vi "PWM舵机驱动实验--基于EIO节点.vi"() -> ()   [LabVIEW 2011]
uses:
  <vilib>/STM32_DriverVI_Interface_F4/PWM-EIO/PWM_Control_F4.ctl
  <vilib>/eio/EIO_TerminalDirection.ctl
  D:/National Instruments/LabVIEW 2011/Targets/Keil/Embedded/RealView/Generic/My_ARM_Starter_Board_F4/STM32_DriverVI_Interface/PWM-EIO/PWM_Channel_16_F4.ctl
  <vilib>/STM32_DriverVI_Interface_F4/Timer/TIM4_Group_Pins_F4.ctl
  <vilib>/STM32_DriverVI_Interface_F4/Timer/TIM4_Channels_Pin_Map_F4.ctl
  <vilib>/STM32_DriverVI_Interface_F4/Timer/TimerX Init_F4.vi
  <vilib>/STM32_DriverVI_Interface_F4/Timer/TIM4 Init_F4.vi
  <vilib>/STM32_DriverVI_Interface_F4/Timer/TimerX Channel Pin Map.vi
  <vilib>/STM32_DriverVI_Interface_F4/Timer/TIM4 Channel Pin Map_F4.vi
  <vilib>/STM32_DriverVI_Interface_F4/Timer/TimerX PWM Mode Set_F4.vi
  <vilib>/STM32_DriverVI_Interface_F4/Timer/TIM4 PWM Mode Set_F4.vi
  <vilib>/STM32_DriverVI_Interface_F4/Timer/TimerX PWM Permit_UnPermit_F4.vi
  <vilib>/STM32_DriverVI_Interface_F4/Timer/TIM4 PWM Permit_UnPermit_F4.vi
  <vilib>/STM32_DriverVI_Interface_F4/Timer/TimerX Int Enable_Disable_F4.vi
  <vilib>/STM32_DriverVI_Interface_F4/Timer/TIM4 Int Enable_Disable_F4.vi
  <vilib>/STM32_DriverVI_Interface_F4/Timer/TimerX PWM Update Duty_F4.vi
  <vilib>/STM32_DriverVI_Interface_F4/Timer/TIM4_PWM_Update_Duty_F4.vi
  <vilib>/eio/EIONode/EIONode.xnode
  <vilib>/STM32_DriverVI_Interface_F4/Timer/TIM5_Channels_Pin_Map_F4.ctl
  <vilib>/STM32_DriverVI_Interface_F4/Timer/TIM5_Group_Pins_F4.ctl
  <vilib>/STM32_DriverVI_Interface_F4/Timer/TIM5 Int Enable_Disable_F4.vi
  <vilib>/STM32_DriverVI_Interface_F4/Timer/TIM5_PWM_Update_Duty_F4.vi
  <vilib>/STM32_DriverVI_Interface_F4/Timer/TIM5 Init_F4.vi
  <vilib>/STM32_DriverVI_Interface_F4/Timer/TIM5 Channel Pin Map_F4.vi
  <vilib>/STM32_DriverVI_Interface_F4/Timer/TIM5 PWM Mode Set_F4.vi
  <vilib>/STM32_DriverVI_Interface_F4/Timer/TIM5 PWM Permit_UnPermit_F4.vi
  <vilib>/STM32_DriverVI_Interface_F4/Timer/TIM3_Channels_Pin_Map_F4.ctl
  <vilib>/STM32_DriverVI_Interface_F4/Timer/TIM3_Group_Pins_F4.ctl
  <vilib>/STM32_DriverVI_Interface_F4/Timer/TIM3 Init_F4.vi
  <vilib>/STM32_DriverVI_Interface_F4/Timer/TIM3 PWM Mode Set_F4.vi
  <vilib>/STM32_DriverVI_Interface_F4/Timer/TIM3 PWM Permit_UnPermit_F4.vi
  <vilib>/STM32_DriverVI_Interface_F4/Timer/TIM3 Int Enable_Disable_F4.vi
  <vilib>/STM32_DriverVI_Interface_F4/Timer/TIM3_PWM_Update_Duty_F4.vi
  <vilib>/STM32_DriverVI_Interface_F4/Timer/TIM3 Channel Pin Map_F4.vi
  <vilib>/STM32_DriverVI_Interface_F4/Timer/TIM2_Channels_Pin_Map_F4.ctl
  <vilib>/STM32_DriverVI_Interface_F4/Timer/TIM2_Group_Pins_F4.ctl
  <vilib>/STM32_DriverVI_Interface_F4/Timer/TIM2 Init_F4.vi
  <vilib>/STM32_DriverVI_Interface_F4/Timer/TIM2 PWM Mode Set_F4.vi
  <vilib>/STM32_DriverVI_Interface_F4/Timer/TIM2 PWM Permit_UnPermit_F4.vi
  <vilib>/STM32_DriverVI_Interface_F4/Timer/TIM2 Int Enable_Disable_F4.vi
  <vilib>/STM32_DriverVI_Interface_F4/Timer/TIM2_PWM_Update_Duty_F4.vi
  <vilib>/STM32_DriverVI_Interface_F4/Timer/TIM2 Channel Pin Map_F4.vi
panel:
  in  "停止":bool
  out "数值":i32
  in  "PWM Enable?":bool
  in  "仪表":u8(knob) scale=0.0..180.0
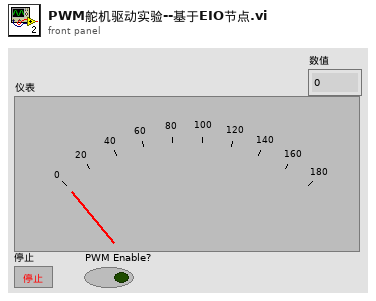
[diagram p1: front panel]
types:
  T1 = typedef "PWM_Control_F4.ctl" = cluster{"Duty(%)":dbl, "PWM Enable?":bool}
  T2 = typedef "波形重生成方式_F4.ctl" = enum8{"写入时立刻重载", "发生更新中断时重载"}
  T3 = typedef "PWM波形形状_F4.ctl" = enum16{"First Low Then High", "First High Then Low"}
  T4 = typedef "PWM输出模式_F4.ctl" = enum8{"Push-pull Output", "Open-drain Output"}
  T5 = typedef "PWM_Channel_16_F4.ctl" = enum8{"PWM_Channel_0", "PWM_Channel_1", "PWM_Channel_2", "PWM_Channel_3", "PWM_Channel_4", "PWM_Channel_5", "PWM_Channel_6", "PWM_Channel_7", "PWM_Channel_8", "PWM_Channel_9", "PWM_Channel_10", "PWM_Channel_11", "PWM_Channel_12", "PWM_Channel_13", "PWM_Channel_14", "PWM_Channel_15"}
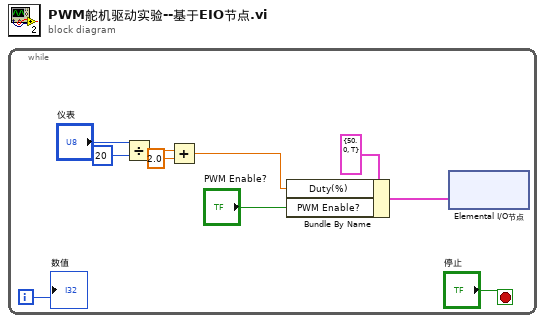
[diagram p0: block diagram]
diagram:
  n1 = while {
    i -> [w3]
    stop <- "停止" stop-if-true
    n2 = Divide(x="仪表", y=u8 20) -> (x/y=w7:dbl)
    n3 = Add(x=w7, y=2.0) -> (x+y=w5:dbl)
    n4 = Bundle By Name(cluster=T1 {"Duty(%)"=50.0, "PWM Enable?"=TRUE} ("Motor"), "Duty(%)"=w5, "PWM Enable?"="PWM Enable?") -> (w1:T1)
    n5 = xnode "Elemental I/O节点"("Motor"=w1) -> ()  [unwired: 1 in, 1 out]
    "数值" <- w3
  }
